vi "GV-file-decode.vi"(1 "string input":string, 2 "offset":i32) -> (0 "string output":string)   [LabVIEW 2020]
doc: "Decode file (into ASCII)"
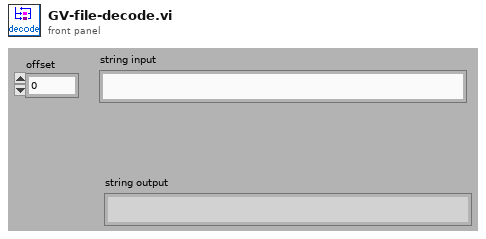
[diagram p1: front panel]
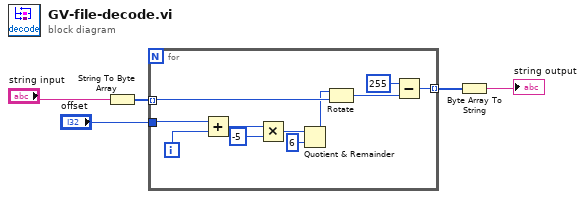
[diagram p0: block diagram]
diagram:
  n1 = String To Byte Array(string="string input") -> (unsigned byte array=w1:u8[])
  n2 = for {
    tunnel: "offset" -> [w16]
    tunnel: w1 -> [w9] mode=indexing
    tunnel: [w6] -> w4 mode=indexing
    i -> [w15]
    n3 = Add(x=w16, y=w15) -> (x+y=w13:i32)
    n4 = Multiply(x=w13, y=-5) -> (x*y=w11:i32)
    n5 = Quotient & Remainder(x=w11, y=6) -> (x-y*floor(x/y)=w8:i32)  [unwired: 1 out]
    n6 = Rotate(1:w9, 2:w8) -> (0:w7:u8)
    n7 = Subtract(x=u8 255, y=w7) -> (x-y=w6:u8)
  }
  n8 = Byte Array To String(unsigned byte array=w4) -> (string=→"string output":string)
